vi "Setting Read Write.vi"(6 "Read/Write":enum16{"Read", "Write"}(ring), 7 "Select":T1, 8 "error in (no error)":errorcluster caption="에러 입력(에러 없음)", 9 "Data in":string[][](array[string])) -> (0 "error out":errorcluster caption="에러 출력", 1 "Data out":string[][](array[string]))   [LabVIEW 2020]
uses:
  Controls/Cmd_Select Setting.ctl
  Controls/Cmd_File Type.ctl
  Controls/Cmd_File path.ctl
  Variables/Global_Cal Info.vi
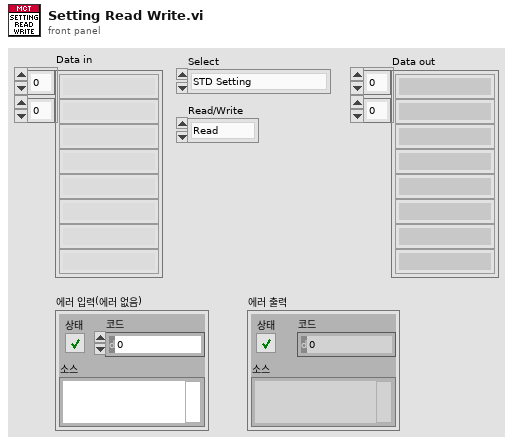
[diagram p1: front panel]
types:
  T1 = typedef "Cmd_Select Setting.ctl" = enum16{"STD Setting"}
  T2 = typedef "Cmd_File path.ctl" = enum16{"에러로그", "데이터파일경로", "성적서원본", "지난성적서", "Data Files", "경로생성", "Updater", "Template", "설정파일경로", "FTP Upload", "Update 경로", "어플리케이션"}
  T3 = typedef "Cmd_File Type.ctl" = enum16{"엑셀", "엑셀(2003)", "텍스트", "설정", "2진", "VI", "CSV", "LOG", "폴더"}
  T4 = typedef "Clst_Cal Info Global.ctl" = cluster{"등록번호":string, "의뢰기관":string, "기기명":string, "제작회사":string, "형식":string, "기기번호":string, "소분류코드":string, "세부분류코드":string, "교정주기":string, "접수번호":string, "교정일자":string, "교정절차서 1":string, "교정절차서 2":string, "교정절차서 3":string, "접수확인자":string, "인증교정자":string, "기술책임자":string, "KOLAS 유무":string, "진행상태":string, "의뢰기관코드":string, "입고형태":string, "영문성적서?":bool, "합불판정?":bool, "부록?":bool, "절차서번호 1":string, "절차서번호 2":string, "절차서번호 3":string, "교정방식":string, "부서명":string}
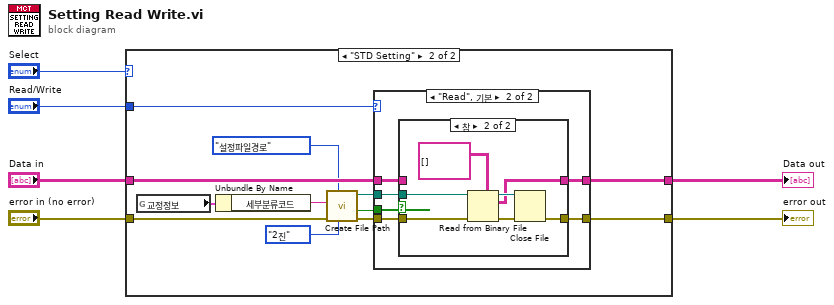
[diagram p0: block diagram]
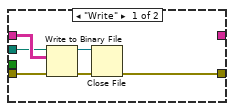
[diagram p3: hidden frame]
diagram:
  n1 = case shown="\"STD Setting\"" "Select" {
    tunnel: "error in (no error)" -> [w7 w8]
    tunnel: [w7 w19] -> w4
    tunnel: "Read/Write" -> [_ w16]
    tunnel: "Data in" -> [_ w18]
    tunnel: [_ w15] -> w1
    frame Default {
    }
    frame "STD Setting" {
      n2 = global read "Global_Cal Info.vi" "교정정보"() -> (w17:T4)
      n3 = Unbundle By Name(w17) -> ("세부분류코드"=w14:string)
      n4 = call "Create File Path.vi"("파일타입"=Cmd_File_Type."2진", "항목"=Cmd_File_path."설정파일경로", "에러 입력"=w8, "문자열 in"=w14) -> ("error out"=w9:errorcluster, "파일존재?"=w10:bool, "파일경로"=w11:path)  [unwired: 4 in, 1 out]
      n5 = case shown="\"Read\", 기본" w16 {
        tunnel: w9 -> [w23 w27]
        tunnel: [w25 w31] -> w19
        tunnel: w18 -> [w24 w30]
        tunnel: w11 -> [w22 w26]
        tunnel: [_ w29] -> w15
        tunnel: w10 -> [_ w28]
        frame "Write" {
          n6 = Write to Binary File(file (use dialog)=w22, data=w24, error in=w23) -> (refnum out=w20:refnum<file>, error out=w21:errorcluster)  [unwired: 3 in, 1 out]
          n7 = Close File(refnum=w20, error in=w21) -> (error out=w25:errorcluster)  [unwired: 1 out]
        }
        frame "Read", Default {
          n8 = case shown="참" w28 {
            tunnel: [w32 w38] -> w31
            tunnel: w30 -> [_ _]
            tunnel: w26 -> [_ w36]
            tunnel: w27 -> [w32 w35]
            tunnel: [_ w34] -> w29
            frame False {
            }
            frame True {
              n9 = Read from Binary File(5:string[][] [], 8:w35, 11:w36) -> (0:w39:errorcluster, 2:w34:string[][], 3:w37:refnum<file>)  [unwired: 3 in, 1 out]
              n10 = Close File(refnum=w37, error in=w39) -> (error out=w38:errorcluster)  [unwired: 1 out]
            }
          }
        }
      }
    }
  }
  "error out" <- w4
  "Data out" <- w1
